vi "RangeFinder.vi"() -> ()   [LabVIEW 2018]
uses:
  <vilib>/myRIO/Instrument Drivers/Onboard IO/AI/typedefs/AI Reference.ctl
  <vilib>/myRIO/Common/Instrument Driver Framework/Utilities/typedefs/myRIO Generic Hardware Reference.ctl
  <vilib>/myRIO/Common/Instrument Driver Framework/Utilities/typedefs/Hardware Version Enum.ctl
  <vilib>/myRIO/Common/Instrument Driver Framework/Utilities/typedefs/myRIO v1.0 Reference.ctl
  <vilib>/myRIO/Common/Instrument Driver Framework/Utilities/typedefs/Generic FPGA Reference.ctl
  <vilib>/myRIO/Common/Instrument Driver Framework/myRIO v1.0/AI/typedefs/AI Channels List.ctl
  <vilib>/myRIO/Common/Instrument Driver Framework/myRIO v1.0/AI/typedefs/AI Channels Enum.ctl
  <vilib>/myRIO/Common/Instrument Driver Framework/Utilities/typedefs/Analog Scaling Constants List.ctl
  <vilib>/myRIO/Common/Instrument Driver Framework/Utilities/typedefs/Analog Scaling Constants.ctl
  <vilib>/userdefined/High Color/nirio_resource_hc.ctl
  <vilib>/myRIO/Common/Instrument Driver Framework/Utilities/vis/Is FPGA Ref Available.vi
  <vilib>/myRIO/Common/Instrument Driver Framework/myRIO v1.0/AI/vis/myRIO v1.1 Open AI.vi
  <vilib>/myRIO/Instrument Drivers/Onboard IO/AI/vis/Read.vi
  <vilib>/Analysis/coordinate.llb/2D Cartesian Coordinate Rotation (Scalar).vi
  <vilib>/Analysis/coordinate.llb/2D Cartesian Coordinate Shift (Scalar).vi
  <vilib>/myRIO/Common/Instrument Driver Framework/Utilities/vis/Validate Channels.vi
  <vilib>/myRIO/Common/Instrument Driver Framework/myRIO v1.0/AI/vis/myRIO v1.0 Reserve AI.vi
  <vilib>/myRIO/Common/Instrument Driver Framework/myRIO v1.0/AI/vis/myRIO v1.0 Build MUX Configuration AI.vi
  <vilib>/myRIO/Common/Instrument Driver Framework/myRIO v1.0/Resource Manager/vis/myRIO v1.0 Reserve Channel List.vi
  <vilib>/myRIO/Common/Instrument Driver Framework/myRIO v1.0/Resource Manager/vis/myRIO v1.0 Reserve Channel.vi
  <vilib>/myRIO/Common/Instrument Driver Framework/myRIO v1.0/Resource Manager/vis/myRIO v1.0 Unreserve Channel.vi
  <vilib>/myRIO/Common/Instrument Driver Framework/myRIO v1.0/Resource Manager/vis/myRIO v1.0 Build Mutex Name.vi
  <vilib>/Utility/VariantDataType/GetNumericInfo.vi
  <vilib>/Utility/error.llb/Error Cluster From Error Code.vi
  <vilib>/myRIO/Common/Instrument Driver Framework/myRIO v1.0/myRIO v1.1 Open.vi
  <vilib>/myRIO/Common/Instrument Driver Framework/myRIO v1.0/AI/vis/myRIO v1.0 Get Scaling Constants AI.vi
  <vilib>/myRIO/Common/Instrument Driver Framework/Utilities/vis/IO Manager.vi
  <vilib>/myRIO/Common/Instrument Driver Framework/Utilities/vis/Configuration Manager.vi
  <vilib>/myRIO/Common/Instrument Driver Framework/myRIO v1.0/myRIO v1.0 Close.vi
  <vilib>/myRIO/Common/Instrument Driver Framework/myRIO v1.0/AI/vis/myRIO v1.0 Read AI.vi
  <vilib>/myRIO/Express VI/Onboard IO/AI/AI Express VI.xnode
  <vilib>/myRIO/Instrument Drivers/Onboard IO/AI/vis/myRIO AI Open.xnode
  <vilib>/ptbypt/NI_PtbyPt.lvlib
  <vilib>/myRIO/Instrument Drivers/Onboard IO/AI/AI.lvlib
  <vilib>/Analysis/NI_AALPro.lvlib
panel:
  in  "Theta":dbl
  in  "Right Arm":bool
  out "Range [cm]":dbl(knob) scale=0.0..80.0
  out "Vo [V]":dbl format="%.2f"
  in  "Kscale [cm-V]":dbl=27.5
  in  "Koffset [cm]":dbl
  out "numeric":dbl format="%_3g"
  in  "Go Left":bool
  out "Position":cluster{"X":dbl, "Y":dbl, "Theta":dbl}
types:
  T1 = typedef "AI.lvlib/AI Reference.ctl" = cluster{"myRIO Reference":T2, "AI Channels List":T6, "AI Scaling Constants List":T8}
  T2 = typedef "myRIO Generic Hardware Reference.ctl" = cluster{"myRIO Model":T3, "myRIO Hardware Reference":T4}
  T3 = typedef "Hardware Version Enum.ctl" = enum16{"Unknown", "myRIO-1900", "myRIO-1950", "roboRIO", "NI ELVIS RIO CM", "ELVIS III"}
  T4 = typedef "myRIO v1.0 Reference.ctl" = cluster{"Generic FPGA Reference":T5, "Allow multiple opens":bool}
  T5 = typedef "Generic FPGA Reference.ctl" = refnum<k20>
  T6 = typedef "AI Channels List.ctl" = T7[]
  T7 = typedef "AI Channels Enum.ctl" = enum16{"Not Connected", "AudioIn/Left", "AudioIn/Right", "C/AI0", "C/AI1", "A/AI0", "A/AI1", "A/AI2", "A/AI3", "A/AI4", "A/AI5", "A/AI6", "A/AI7", "B/AI0", "B/AI1", "B/AI2", "B/AI3", "B/AI4", "B/AI5", "B/AI6", "B/AI7", "AI/AI0", "AI/AI1", "AI/AI2", "AI/AI3", "A/AI0 (DIFF)", "A/AI1 (DIFF)", "A/AI2 (DIFF)", "A/AI3 (DIFF)", "B/AI0 (DIFF)", "B/AI1 (DIFF)", "B/AI2 (DIFF)", "B/AI3 (DIFF)"}
  T8 = typedef "Analog Scaling Constants List.ctl" = T9[]
  T9 = typedef "Analog Scaling Constants.ctl" = cluster{"LSB Weight (Volts)":dbl, "Offset (Volts)":dbl, "Signed?":bool}
  T10 = typedef "nirio_resource_hc.ctl" = tag
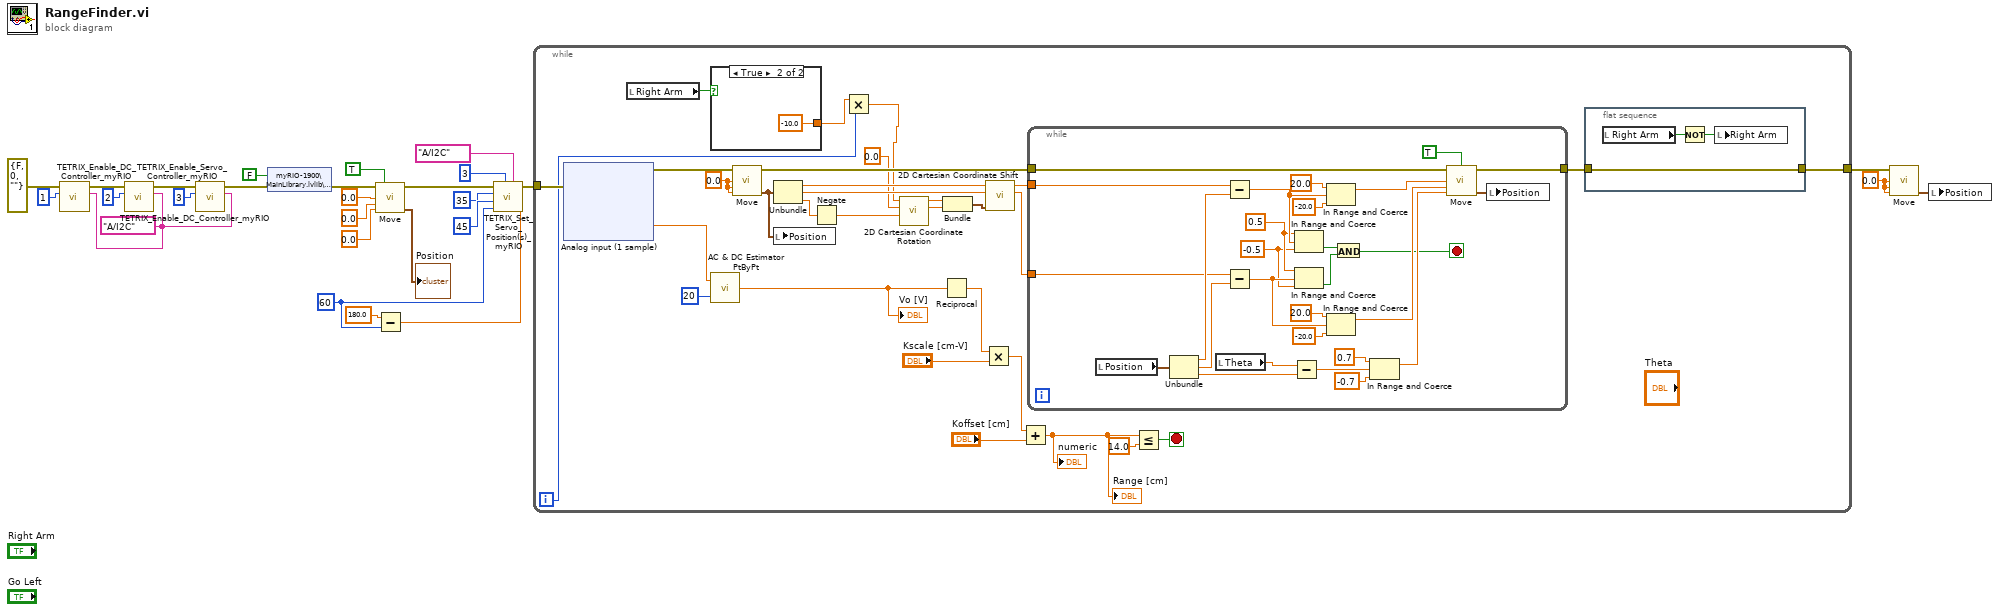
[diagram p0: block diagram]
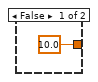
[diagram p2: hidden frame]
diagram:
  w2 = 0.0 ("x (mm/s)")
  w5 = tag "A/I2C" ("myRIO MXP Port A/B")
  w15 = u8 60 ("Servo 4 Position (0 - 180 degrees)")
  n1 = call <vilib>:"TETRIX_Enable_DC_Controller_myRIO.vi"("myRIO MXP Port A/B"=w5, "Controller ID#  (I2C Address)"=u8 1, "Error/Flow In"=errorcluster {"status"=FALSE, "code"=0, "source"=""}) -> ("Error/Flow Out"=w27:errorcluster)  [unwired: 4 in]
  n2 = call <vilib>:"TETRIX_Enable_DC_Controller_myRIO.vi"("myRIO MXP Port A/B"=w5, "Controller ID#  (I2C Address)"=u8 2, "Error/Flow In"=w27) -> ("Error/Flow Out"=w25:errorcluster)  [unwired: 4 in]
  n3 = call <vilib>:"TETRIX_Enable_Servo_Controller_myRIO.vi"("myRIO MXP Port A/B"=w5, "Controller ID#  (I2C Address)"=u8 3, "Error/Flow In"=w25) -> ("Error/Flow Out"=w24:errorcluster)  [unwired: 4 in]
  n4 = shared-variable "myRIO-1900\\MainLibrary.lvlib\\stop"(FALSE ("Stop"), error in=w24) -> (error out=w22:errorcluster)
  n5 = call "Move.vi"("Error/Flow In"=w22, "Reset"=TRUE, "x (mm/s)"=0.0, "y (mm/s)"=0.0, "theta (rad/s)"=0.0) -> ("Error/Flow Out"=w10:errorcluster, "Position"=→"Position":cluster{"X":dbl, "Y":dbl, "Theta":dbl})  [unwired: 9 in]
  n6 = Subtract(x=180.0, y=w15) -> (x-y=w14:dbl)
  n7 = call <vilib>:"TETRIX_Set_Servo_Position(s)_myRIO.vi"("Servo 4 Position (0 - 180 degrees)"=w14, "myRIO MXP Port A/B"=tag "A/I2C", "Controller ID#  (I2C Address)"=u8 3, "Servo 3 Position (0 - 180 degrees)"=w15, "Servo 2 Position (0 - 180 degrees)"=u8 45, "Servo 1 Position (0 - 180 degrees)"=u8 35 ("Controller ID#  (I2C Address)"), "Error/Flow In"=w10) -> ("Error/Flow Out"=w4:errorcluster)  [unwired: 2 in]
  n8 = while {
    tunnel: w4 -> [w48]
    tunnel: [w31] -> w1
    i -> [w29]
    stop <- w57 stop-if-true
    w34 = 0.0 ("x (mm/s)")
    n9 = xnode "Analog input (1 sample)"("error in (no error)"=w48) -> ("B/AI0 (Pin 3)"=w52:dbl, "error out"=w33:errorcluster)
    n10 = local read "Right Arm"() -> (w45:bool)
    n11 = case shown="True" w45 {
      tunnel: [10.0 -10.0] -> w30
      frame False {
      }
      frame True {
      }
    }
    n12 = call <vilib>:"AC & DC Estimator PtByPt.vi"("signal"=w52, "sample length"=20) -> ("DC estimate (V)"=w53:dbl)  [unwired: 1 in, 2 out]
    "Vo [V]" <- w53
    n13 = call "Move.vi"("Error/Flow In"=w33, "x (mm/s)"=w34, "y (mm/s)"=w34, "theta (rad/s)"=w34) -> ("Error/Flow Out"=w44:errorcluster, "Position"=w35:cluster{"X":dbl, "Y":dbl, "Theta":dbl})  [unwired: 10 in]
    n14 = Unbundle(w35) -> ("X"=w40:dbl, "Y"=w41:dbl, "Theta"=w47:dbl)
    n15 = local write "Position"(w35) -> ()
    n16 = Negate(x=w47) -> (-x=w46:dbl)
    n17 = Multiply(x=w30, y=w29) -> (x*y=w28:dbl)
    n18 = call-poly <vilib>:"2D Cartesian Coordinate Rotation.vi"("theta"=w46, "y"=0.0, "x"=w28) -> ("y out"=w38:dbl, "x out"=w37:dbl)  [unwired: 6 in, 1 out]
    n19 = Reciprocal(x=w53) -> (1/x=w50:dbl)
    n20 = Bundle("x out"=w37, "y out"=w38) -> (w39:cluster{"x out":dbl, "y out":dbl})  [unwired: 1 in]
    n21 = Multiply(x=w50, y="Kscale [cm-V]") -> (x*y=w56:dbl)
    n22 = call-poly <vilib>:"2D Cartesian Coordinate Shift.vi"("shift"=w39, "y"=w41, "x"=w40) -> ("y out"=w43:dbl, "x out"=w42:dbl)  [unwired: 6 in, 1 out]
    n23 = Add(x=w56, y="Koffset [cm]") -> (x+y=w49:dbl)
    "Range [cm]" <- w49
    "numeric" <- w49
    n24 = while {
      tunnel: w42 -> [w89]
      tunnel: w43 -> [w83]
      tunnel: w44 -> [w71]
      tunnel: [w65] -> w32
      stop <- w64 stop-if-true
      w67 = -0.5 ("upper limit")
      w68 = 0.5 ("upper limit")
      n25 = local read "Position"() -> (w91:cluster{"X":dbl, "Y":dbl, "Theta":dbl})
      n26 = Unbundle(w91) -> ("X"=w90:dbl, "Y"=w84:dbl, "Theta"=w82:dbl)
      n27 = local read "Theta"() -> (w66:dbl)
      n28 = Subtract(x=w89, y=w90) -> (x-y=w75:dbl)
      n29 = Subtract(x=w83, y=w84) -> (x-y=w76:dbl)
      n30 = Subtract(x=w66, y=w82) -> (x-y=w81:dbl)
      n31 = In Range and Coerce(upper limit=w68, x=w75, lower limit=w67) -> (In Range?=w77:bool)  [unwired: 1 out]
      n32 = In Range and Coerce(upper limit=w68, x=w76, lower limit=w67) -> (In Range?=w78:bool)  [unwired: 1 out]
      n33 = In Range and Coerce(upper limit=20.0, x=w75, lower limit=-20.0) -> (coerced(x)=w72:dbl)  [unwired: 1 out]
      n34 = In Range and Coerce(upper limit=20.0, x=w76, lower limit=-20.0) -> (coerced(x)=w73:dbl)  [unwired: 1 out]
      n35 = And(x=w77, y=w78) -> (x .and. y?=w64:bool)
      n36 = In Range and Coerce(upper limit=0.7, x=w81, lower limit=-0.7 ("upper limit")) -> (coerced(x)=w74:dbl)  [unwired: 1 out]
      n37 = call "Move.vi"("Error/Flow In"=w71, "Relative to Global Frame"=TRUE, "x (mm/s)"=w72, "y (mm/s)"=w73, "theta (rad/s)"=w74) -> ("Error/Flow Out"=w65:errorcluster, "Position"=w70:cluster{"X":dbl, "Y":dbl, "Theta":dbl})  [unwired: 9 in]
      n38 = local write "Position"(w70) -> ()
    }
    n39 = Less Or Equal?(x=w49, y=14.0) -> (x <= y?=w57:bool)
    n40 = flat-sequence {
      tunnel: w32 -> [w59]
      tunnel: [w59] -> w31
      frame #0 {
        n41 = local read "Right Arm"() -> (w61:bool)
        n42 = Not(x=w61) -> (.not. x?=w60:bool)
        n43 = local write "Right Arm"(w60) -> ()
      }
    }
  }
  n44 = call "Move.vi"("Error/Flow In"=w1, "x (mm/s)"=w2, "y (mm/s)"=w2, "theta (rad/s)"=w2) -> ("Position"=w3:cluster{"X":dbl, "Y":dbl, "Theta":dbl})  [unwired: 10 in, 1 out]
  n45 = local write "Position"(w3) -> ()
